vi "bats.parser.test.AddOrderLong.add.four.orders.vi"(10 "Expected OrderBook.Command[]":T1[](array[typedef])=[{"OrderBook Command.Type"=enum."AddOrder", "Side (U8)"=66, "Order Id (U64)"=3544385890602799695, "Quantity (U32)"=20000, "Symbol (U64)"=4702127773838213120, "Price (U64)"=9050, "Executed Quantity (U32)"=0, "Cancelled Quantity (U32)"=0}, {"OrderBook Command.Type"=enum."AddOrder", "Side (U8)"=66, "Order Id (U64)"=3616443484640727631, "Quantity (U32)"=20000, "Symbol (U64)"=4702127773838213120, "Price (U64)"=9050, "Executed Quantity (U32)"=0, "Cancelled Quantity (U32)"=0}, {"OrderBook Command.Type"=enum."AddOrder", "Side (U8)"=66, "Order Id (U64)"=3688501078678655567, "Quantity (U32)"=20000, "Symbol (U64)"=4702127773838213120, "Price (U64)"=9050, "Executed Quantity (U32)"=0, "Cancelled Quantity (U32)"=0}, {"OrderBook Command.Type"=enum."AddOrder", "Side (U8)"=66, "Order Id (U64)"=3760558672716583503, "Quantity (U32)"=20000, "Symbol (U64)"=4702127773838213120, "Price (U64)"=9050, "Executed Quantity (U32)"=0, "Cancelled Quantity (U32)"=0}] {"Side (U8)" format="%.0x"; "Order Id (U64)" format="%.0x"; "Symbol (U64)" format="%.0x"}, 11 "Test.Messages":T3[](array[typedef])=[{"MessageType"=enum."AddOrderLong", "AddOrderLong.Parms"={"Time Offset"=447000, "Order Id"="ORID0001", "Side Indicator"="B", "Quantity"=20000, "Symbol"="AAPL", "Price"=0.905, "Add Flags"=1}, "Time.Parms"={"Seconds Since Midnight"=447000}, "SequencedUnitHeader.Parms"={"Hdr Count"=32, "Hdr Unit"=1, "Hdr Sequence"=1, "Starting Sequence"=1}}, {"MessageType"=enum."AddOrderLong", "AddOrderLong.Parms"={"Time Offset"=447000, "Order Id"="ORID0002", "Side Indicator"="B", "Quantity"=20000, "Symbol"="AAPL", "Price"=0.905, "Add Flags"=1}, "Time.Parms"={"Seconds Since Midnight"=447000}, "SequencedUnitHeader.Parms"={"Hdr Count"=32, "Hdr Unit"=1, "Hdr Sequence"=1, "Starting Sequence"=1}}, {"MessageType"=enum."AddOrderLong", "AddOrderLong.Parms"={"Time Offset"=447000, "Order Id"="ORID0003", "Side Indicator"="B", "Quantity"=20000, "Symbol"="AAPL", "Price"=0.905, "Add Flags"=1}, "Time.Parms"={"Seconds Since Midnight"=447000}, "SequencedUnitHeader.Parms"={"Hdr Count"=32, "Hdr Unit"=1, "Hdr Sequence"=1, "Starting Sequence"=1}}, {"MessageType"=enum."AddOrderLong", "AddOrderLong.Parms"={"Time Offset"=447000, "Order Id"="ORID0004", "Side Indicator"="B", "Quantity"=20000, "Symbol"="AAPL", "Price"=0.905, "Add Flags"=1}, "Time.Parms"={"Seconds Since Midnight"=447000}, "SequencedUnitHeader.Parms"={"Hdr Count"=32, "Hdr Unit"=1, "Hdr Sequence"=1, "Starting Sequence"=1}}]) -> ()   [LabVIEW 2022 SP3]
uses:
  Message.Spec.ctl
  pitch/MessageType.ctl
  pitch/AddOrderLong/AddOrderLong.Parameters.ctl
  pitch/Time/Time.Parameters.ctl
  pitch/SequencedUnitHeader/SequencedUnitHeader.Parameters.ctl
  arty/orderbook/orderbook.command.ctl
  arty/orderbook/orderbook.command.type.ctl
  pitch/Time/Time.lvclass
  pitch/AddOrderLong/AddOrderLong.lvclass
  pitch/SequencedUnitHeader/SequencedUnitHeader.lvclass
panel:
  in  "Watch.List":string[](array[string])=["AAPL"]
  out "Passed":bool
  out "Results":T1[](array[typedef]) {"Side (U8)" format="%.0x"; "Order Id (U64)" format="%.0x"; "Symbol (U64)" format="%.0x"}
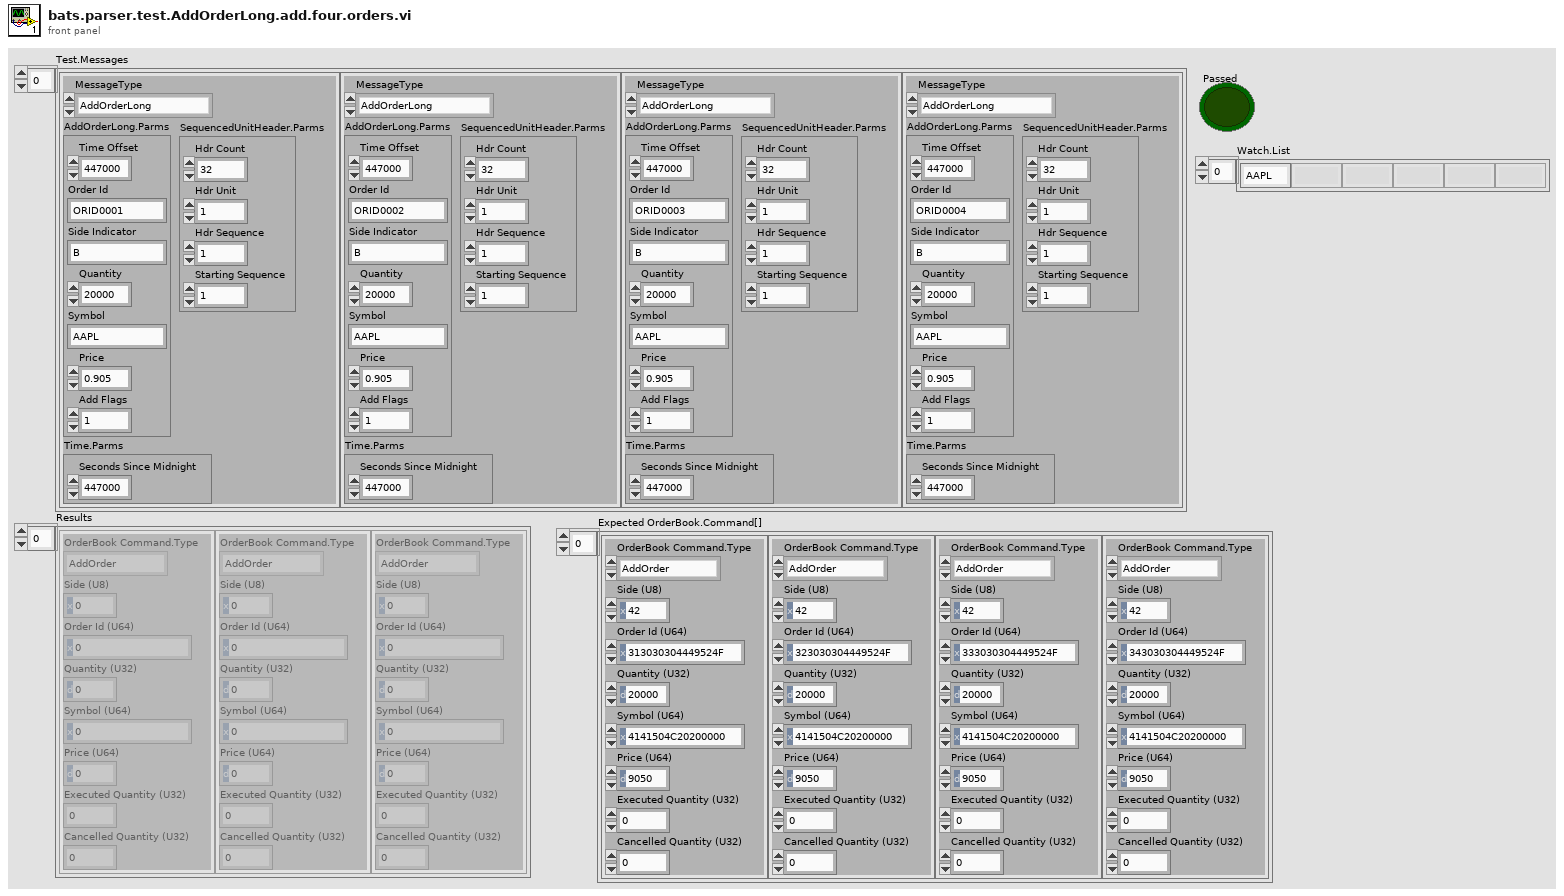
[diagram p1: front panel]
types:
  T1 = typedef "orderbook.command.ctl" = cluster{"OrderBook Command.Type":T2, "Side (U8)":u8, "Order Id (U64)":u64, "Quantity (U32)":u32, "Symbol (U64)":u64, "Price (U64)":u64, "Executed Quantity (U32)":u32, "Cancelled Quantity (U32)":u32}
  T2 = typedef "orderbook.command.type.ctl" = enum16{"AddOrder", "OrderExecuted", "ReduceSize", "ModifyOrder", "DeleteOrder", "Get.All.Orders", "Get.Top"}
  T3 = typedef "Message.Spec.ctl" = cluster{"MessageType":T4, "AddOrderLong.Parms":T5, "Time.Parms":T6, "SequencedUnitHeader.Parms":T7}
  T4 = typedef "MessageType.ctl" = enum16{"SequencedUnitHeader", "AddOrderLong", "AddOrderShort", "AddOrderExpanded", "Time"}
  T5 = typedef "AddOrderLong.lvclass/AddOrderLong.Parameters.ctl" = cluster{"Time Offset":u32, "Order Id":string, "Side Indicator":string, "Quantity":u32, "Symbol":string, "Price":dbl, "Add Flags":u8}
  T6 = typedef "Time.lvclass/Time.Parameters.ctl" = cluster{"Seconds Since Midnight":u32}
  T7 = typedef "SequencedUnitHeader.lvclass/SequencedUnitHeader.Parameters.ctl" = cluster{"Hdr Count":u8, "Hdr Unit":u8, "Hdr Sequence":u32, "Starting Sequence":u32}
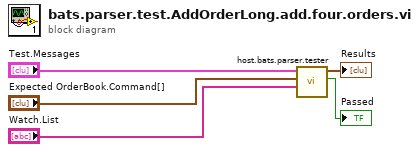
[diagram p0: block diagram]
diagram:
  n1 = call "host.bats.parser.tester.vi"("Watch.List"="Watch.List", "Expected OrderBook.Command[]"="Expected OrderBook.Command[]", "Test.Messages"="Test.Messages") -> ("Passed"=→"Passed":bool, "OrderBook.Command[]"=→"Results":T1[])  [unwired: 5 in, 2 out]
